vi "Simulador.vi"(8 "error in (no error)":errorcluster, 10 "amplitud":dbl, 11 "frecuencia":dbl) -> (0 "error out":errorcluster, 2 "amp out":dbl, 3 "frec out":dbl)   [LabVIEW 2019, in "Prueba.lvclass"]
uses:
  Prueba.lvclass
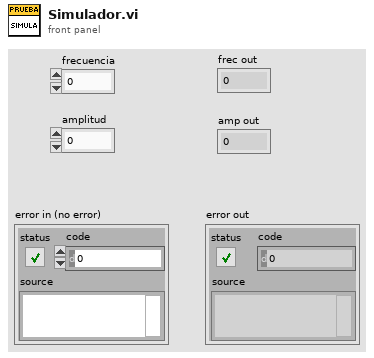
[diagram p1: front panel]
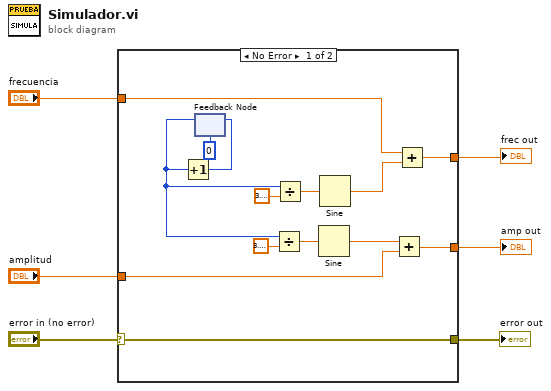
[diagram p0: block diagram]
diagram:
  n1 = case shown="No Error" "error in (no error)" {
    selector: "error in (no error)" -> [w7 w21]
    tunnel: "frecuencia" -> [w17 _]
    tunnel: [w16 _] -> w5
    tunnel: "amplitud" -> [w10 _]
    tunnel: [w9 _] -> w3
    tunnel: [w7 w21] -> w1
    frame No Error {
      n2 = feedback #1(0) -> (w8:i32)
      n3 = Increment(x=w8) -> (x+1=w15:i32)
      n4 = feedback-in #1(w15) -> ()
      n5 = Divide(x=w8, y=3.141592653589793) -> (x/y=w13:dbl)
      n6 = Divide(x=w8, y=3.141592653589793) -> (x/y=w18:dbl)
      n7 = Sine(x=w13) -> (sin(x)=w11:dbl)
      n8 = Sine(x=w18) -> (sin(x)=w20:dbl)
      n9 = Add(x=w11, y=w10) -> (x+y=w9:dbl)
      n10 = Add(x=w17, y=w20) -> (x+y=w16:dbl)
    }
    frame Error {
    }
  }
  "frec out" <- w5
  "amp out" <- w3
  "error out" <- w1
